vi "Define Folder Exclusion List.vi"(8 "error in (no error)":errorcluster, 11 "File Explorer in":refnum<class "File Explorer.lvclass">) -> (0 "error out":errorcluster, 3 "File Explorer out":refnum<class "File Explorer.lvclass">)   [LabVIEW 2020, in "File Explorer.lvlib" / "File Explorer.lvclass"]
uses:
  <vilib>/gpm_packages/@cs/file-explorer-extension/Source/File Explorer/File Explorer/File Explorer.lvclass
  <vilib>/gpm_packages/@cs/file-explorer-extension/Source/File Explorer/File Explorer/File Explorer.lvclass/File Explorer.ctl
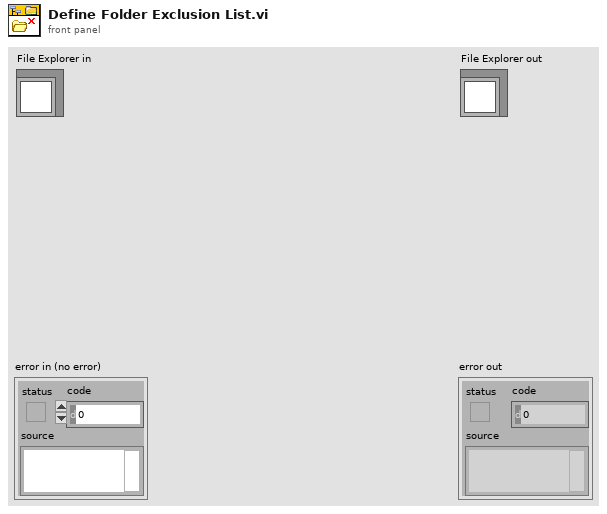
[diagram p1: front panel]
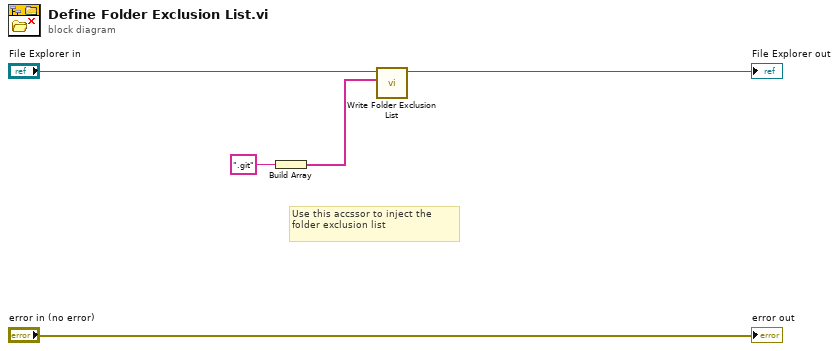
[diagram p0: block diagram]
diagram:
  # "Use this accssor to inject the\nfolder exclusion list"
  n1 = Build Array(".git") -> (w1:string[])
  n2 = call <vilib>:"Write Folder Exclusion List.vi"("Folder Exclusion List"=w1, "File Explorer in"="File Explorer in") -> ("File Explorer out"=→"File Explorer out":refnum<class "File Explorer.lvclass">)  [unwired: 9 in]
  "error out" <- "error in (no error)"
